vi "Populate Type Map.vi"(8 "error in (no error)":errorcluster, 11 "TwinCAT ADS in":refnum<class "TwinCAT ADS.lvclass">) -> (0 "error out":errorcluster, 3 "TwinCAT ADS out":refnum<class "TwinCAT ADS.lvclass">)   [LabVIEW 2018, in "TwinCAT ADS.lvclass"]
uses:
  TwinCAT ADS.lvclass
  TwinCAT ADS.lvclass/TwinCAT ADS.ctl
  TwinCAT.Ads
  Get Type Map.vi
  <vilib>/Utility/error.llb/Trim Whitespace.vi
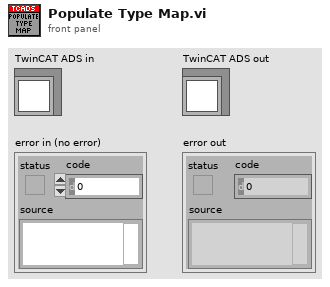
[diagram p1: front panel]
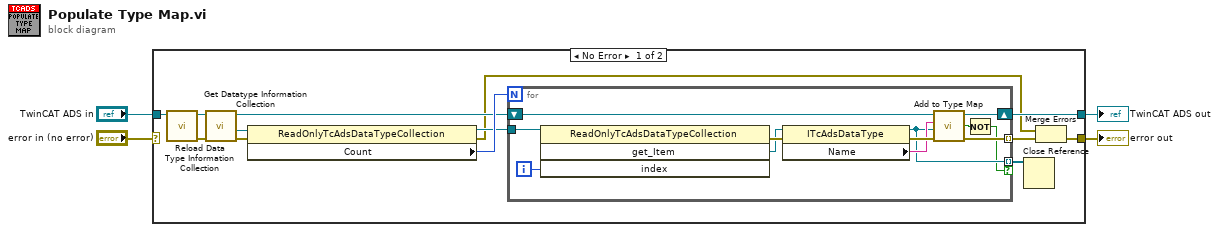
[diagram p0: block diagram]
diagram:
  n1 = case shown="No Error" "error in (no error)" {
    selector: "error in (no error)" -> [_ w31]
    tunnel: "TwinCAT ADS in" -> [w14 w30]
    tunnel: [w6 w31] -> w1
    tunnel: [w15 w30] -> w2
    frame No Error {
      n2 = call "Reload Data Type Information Collection.vi"("TwinCAT ADS in"=w14) -> ("error out"=w12:errorcluster, "TwinCAT ADS out"=w13:refnum<class "TwinCAT ADS.lvclass">)  [unwired: 9 in]
      n3 = call "Get Datatype Information Collection.vi"("error in (no error)"=w12, "TwinCAT ADS in"=w13) -> ("error out"=w10:errorcluster, ".NET AdsDatatypeInfoCollection"=w8:refnum<k24>, "TwinCAT ADS out"=w11:refnum<class "TwinCAT ADS.lvclass">)  [unwired: 7 in]
      n4 = property class="ReadOnlyTcAdsDataTypeCollection"(reference=w8, error in=w10) -> (reference out=w16:refnum<k24>, error out=w5:errorcluster, "Count"=w17:i32)
      n5 = for {
        N: w17 -> [_]
        tunnel: w16 -> [w29]
        shift-right: [w22] -> w15
        shift-left: w11 -> [w23]
        tunnel: [w24] -> w9 mode=indexing
        tunnel: [w20] -> w7 mode=indexing if=w18
        i -> [w26]
        n6 = invoke class="ReadOnlyTcAdsDataTypeCollection" method="get_Item"(reference=w29, "index"=w26) -> (error out=w28:errorcluster, "get_Item"=w27:refnum<k24>)  [unwired: 2 in, 2 out]
        n7 = property class="ITcAdsDataType"(reference=w27, error in=w28) -> (reference out=w20:refnum<k24>, error out=w25:errorcluster, "Name"=w21:string)
        n8 = call "Add to Type Map.vi"("error in (no error)"=w25, ".NET AdsDataType"=w20, "Type Name"=w21, "TwinCAT ADS in"=w23) -> ("error out"=w24:errorcluster, "Success?"=w19:bool, "TwinCAT ADS out"=w22:refnum<class "TwinCAT ADS.lvclass">)  [unwired: 5 in]
        n9 = Not(x=w19) -> (.not. x?=w18:bool)
      }
      n10 = Close Reference(reference=w7) -> ()  [unwired: 1 in, 1 out]
      n11 = Merge Errors(w5, w9) -> (w6:errorcluster)
    }
    frame Error {
    }
  }
  "error out" <- w1
  "TwinCAT ADS out" <- w2
